vi "Read Child Attributes.vi"(11 "Actor in":refnum<class "Actor.lvclass">) -> (2 "Child Attributes":T1)   [LabVIEW 2020, in "jettl.lvlib" / "Actor.lvclass"]
uses:
  Actor.lvclass
  Msg/Msg.lvclass
  Transport/Transport.lvclass
  Attributes Metadata/Attributes Metadata.lvclass
  Child Attributes.ctl
  jettl.lvlib
  Msgs.ctl
  Attributes.ctl
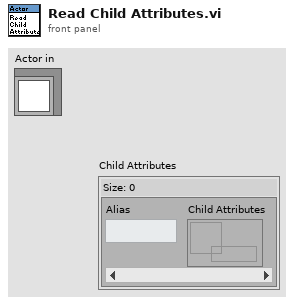
[diagram p1: front panel]
types:
  T1 = typedef "jettl.lvlib/Child Attributes.ctl" = map{string, refnum<data-value>}
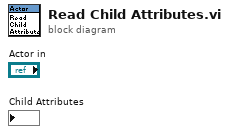
[diagram p0: block diagram]
diagram:
